vi "Register XNET Database.vi"(8 "error in (no error)":errorcluster, 10 "alias":string, 11 "database path":path) -> (0 "error out":errorcluster, 2 "alias":string)   [LabVIEW 2017]
uses:
  <userlib>/_OpenG.lib/file/file.llb/Strip Path Extension - String__ogtk.vi
  <userlib>/_OpenG.lib/file/file.llb/Append Path to Root if Relative - Scalar__ogtk.vi
  niveristand-custom-device-testing-tools/VeriStandTestUtilities/VeriStandTestUtilities.lvlib
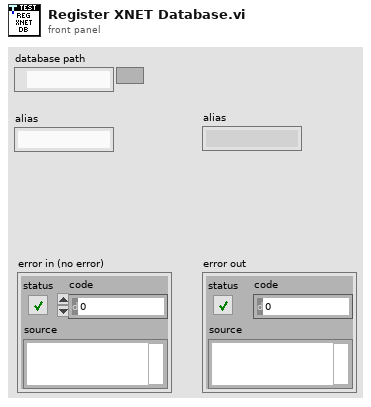
[diagram p1: front panel]
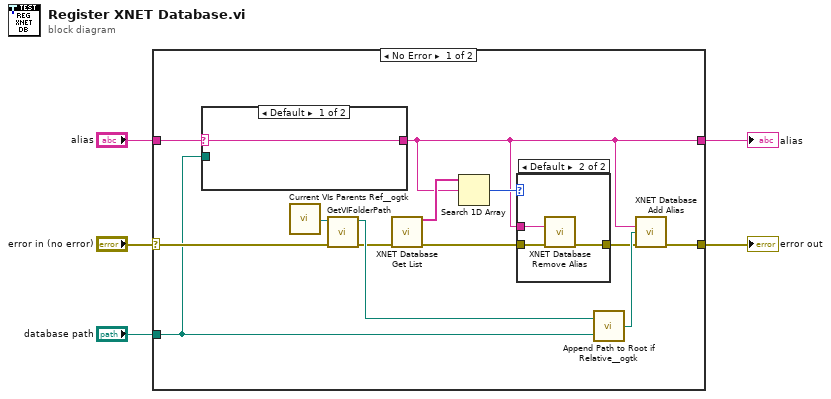
[diagram p0: block diagram]
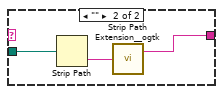
[diagram p2: hidden frame]
diagram:
  n1 = case shown="No Error" "error in (no error)" {
    selector: "error in (no error)" -> [w9 w27]
    tunnel: [w16 w27] -> w5
    tunnel: "alias" -> [w8 _]
    tunnel: "database path" -> [w7 _]
    tunnel: [w6 _] -> w1
    frame No Error {
      n2 = case shown="Default" w8 {
        selector: w8 -> [w19 _]
        tunnel: [w19 w21] -> w6
        tunnel: w7 -> [_ w22]
        frame Default {
        }
        frame "" {
          n3 = Strip Path(path=w22) -> (name=w20:string)  [unwired: 1 out]
          n4 = call-poly <userlib>:"Strip Path Extension__ogtk.vi"("path"=w20) -> ("root"=w21:string)  [unwired: 1 out]
        }
      }
      n5 = call <userlib>:"Current VIs Parents Ref__ogtk.vi"() -> ("Calling VI's Reference"=w11:refnum<vi>)  [unwired: 2 in]
      n6 = call "GetVIFolderPath.vi"("error in (no error)"=w9, "VI Reference in"=w11) -> ("error out"=w10:errorcluster, "VI Folder Path out"=w17:path)  [unwired: 8 in]
      n7 = call <vilib>:"XNET Database Get List.vi"("error in (no error)"=w10) -> ("array of alias"=w12:string[], "error out"=w14:errorcluster)  [unwired: 12 in, 1 out]
      n8 = Search 1D Array(1D array=w12, element=w6) -> (index of element=w13:i32)  [unwired: 1 in]
      n9 = case shown="Default" w13 {
        tunnel: w14 -> [w23 w26]
        tunnel: [w23 w25] -> w15
        tunnel: w6 -> [_ w24]
        frame -1 {
        }
        frame Default {
          n10 = call <vilib>:"XNET Database Remove Alias.vi"("alias"=w24, "error in (no error)"=w26) -> ("error out"=w25:errorcluster)  [unwired: 13 in]
        }
      }
      n11 = call-poly <userlib>:"Append Path to Root if Relative__ogtk.vi"("Absolute or Relative Path"=w7, "Root Path"=w17) -> ("Absolute or Appended Path"=w18:path)
      n12 = call <vilib>:"XNET Database Add Alias.vi"("alias"=w6, "filepath"=w18, "error in (no error)"=w15) -> ("error out"=w16:errorcluster)  [unwired: 12 in]
    }
    frame Error {
    }
  }
  "error out" <- w5
  "alias" <- w1
